vi "PickedObjects.vi"(8 "error in (no error)":errorcluster, 10 "Point":T1, 11 "Render Window in":refnum<class "Render Window.lvclass">) -> (0 "error out":errorcluster, 2 "Objects":refnum<class "3D Object.lvclass">[](array[class]), 3 "Render Window out":refnum<class "Render Window.lvclass">)   [LabVIEW 2015, in "Render Window.lvclass"]
uses:
  Render Window.lvclass
  <vilib>/Utility/miscctls.llb/LVPoint32TypeDef.ctl
  3D Object/3D Object.lvclass
  Render Window.lvclass/Render Window.ctl
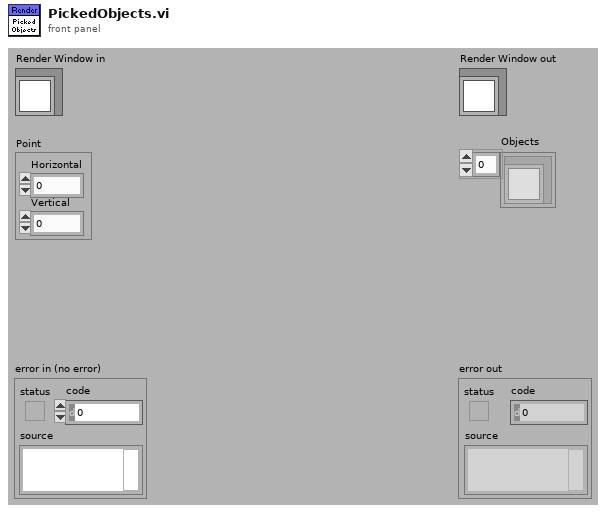
[diagram p1: front panel]
types:
  T1 = typedef "LVPoint32TypeDef.ctl" = cluster{"Horizontal":i32, "Vertical":i32}
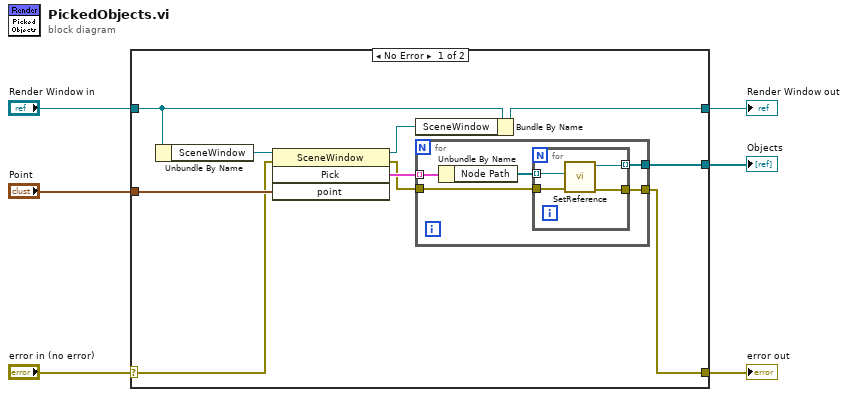
[diagram p0: block diagram]
diagram:
  n1 = case shown="No Error" "error in (no error)" {
    selector: "error in (no error)" -> [w13 w27]
    tunnel: [w8 w27] -> w5
    tunnel: [w10 w26] -> w3
    tunnel: "Render Window in" -> [w11 w26]
    tunnel: "Point" -> [w15 _]
    tunnel: [w7 _] -> w1
    frame No Error {
      n2 = Unbundle By Name(w11) -> ("SceneWindow"=w16:refnum<vi>)
      n3 = invoke class="SceneWindow" method="Pick"(reference=w16, error in=w13, "point"=w15) -> (reference out=w9:refnum<vi>, error out=w12:errorcluster, "Pick"=w14:cluster{"Node Path":refnum<vi>[]}[])  [unwired: 1 in, 1 out]
      n4 = Bundle By Name(cluster=w11, "SceneWindow"=w9) -> (w10:refnum<class "Render Window.lvclass">)
      n5 = for {
        tunnel: w14 -> [w21] mode=indexing
        tunnel: w12 -> [w19]
        tunnel: [w18] -> w8
        tunnel: [w17] -> w7
        n6 = Unbundle By Name(w21) -> ("Node Path"=w20:refnum<vi>[])
        n7 = for {
          tunnel: w20 -> [w25] mode=indexing
          tunnel: w19 -> [w24]
          tunnel: [w23] -> w17 mode=indexing
          tunnel: [w22] -> w18
          n8 = call "SetReference.vi"("error in (no error)"=w24, "SceneObject"=w25) -> ("error out"=w22:errorcluster, "3D Object out"=w23:refnum<class "3D Object.lvclass">)  [unwired: 8 out]
        }
      }
    }
    frame Error {
    }
  }
  "error out" <- w5
  "Render Window out" <- w3
  "Objects" <- w1
